vi "try_Double-Click While Wiring.vi"   [LabVIEW 2020]
panel:
  # "Double-Click While Wiring Demo"
  # "See the block diagram."
  # "Close this VI when you are done with the demo."
  # "You do not need to save changes to this VI."
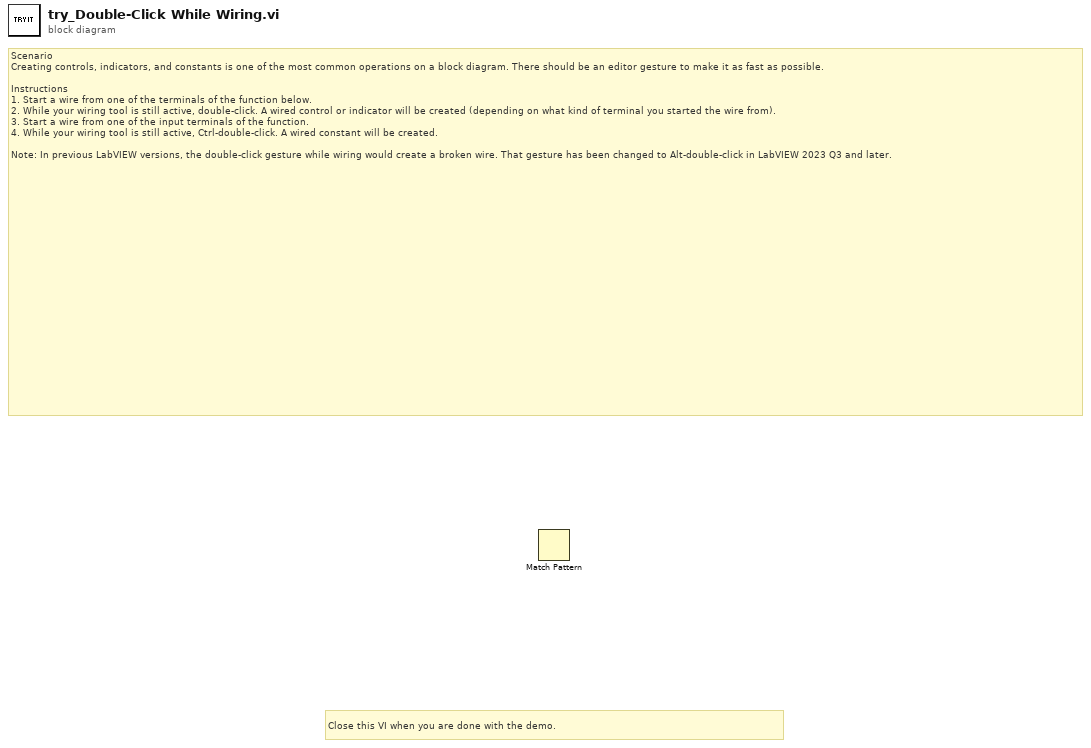
[diagram p0: block diagram]
diagram:
  # "Close this VI when you are done with the demo."
  # "Scenario\nCreating controls, indicators, and constants is one of the most common operations on a block diagram. There should be an editor gesture to make it as fast as possible.\n\nInstructions\n1. Start a wire from one of the terminals of the function below.\n2. While your wiring tool is still active, double-click. A wired control or indicator will be created (depending on what kind of terminal you started the wire from).\n3. Start a wire from one of the input terminals of the function.\n4. While your wiring tool is still active, Ctrl-double-click. A wired constant will be created.\n\nNote: In previous LabVIEW versions, the double-click gesture while wiring would create a broken wire. That gesture has been changed to Alt-double-click in LabVIEW 2023 Q3 and later."
  n1 = Match Pattern() -> ()  [unwired: 3 in, 4 out]
